vi "niRFUtil RFHS Channelizer DesignFilter_BlockSize.vi"(0 "fs":dbl=1.0, 5 "Channel Specification":T1={"fc"=0.0, "fs"=1.0, "passBW"=0.0, "stopBW"=0.0, "Rejection (dB)"=0.0, "Flags"=0, "Reserved"=0} {"Flags" items=["None"=0, "Force Fractional"=1, "Use Multistage"=2, "Use Pretrigger Data "=256, "Frequency Shift Only"=4]; "fs" format="%#_8p"; "fc" format="%#_6p"; "stopBW" format="%#_6p"; "passBW" format="%#_6p"}, 11 "error in (no error)":errorcluster) -> (4 "Filter Taps":i32, 6 "upsample":i32, 8 "downsample":dbl, 15 "error out":errorcluster)   [LabVIEW 2015, in "niRFUtil.lvlib"]
uses:
  niRFUtil.lvlib
  Includes/niRFUtil RFHS Channelizer ChannelSpecificationBase.ctl
  Includes/niRFUtil RFHS Channelizer ChannelFlags.ctl
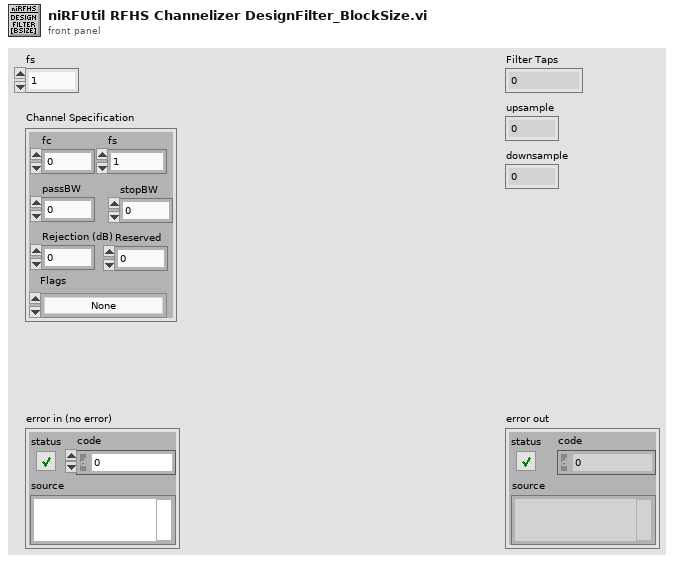
[diagram p1: front panel]
types:
  T1 = typedef "niRFUtil.lvlib/niRFUtil RFHS Channelizer ChannelSpecificationBase.ctl" = cluster{"fc":dbl, "fs":dbl, "passBW":dbl, "stopBW":dbl, "Rejection (dB)":dbl, "Flags":T2, "Reserved":i32}
  T2 = typedef "niRFUtil.lvlib/niRFUtil RFHS Channelizer ChannelFlags.ctl" = u32
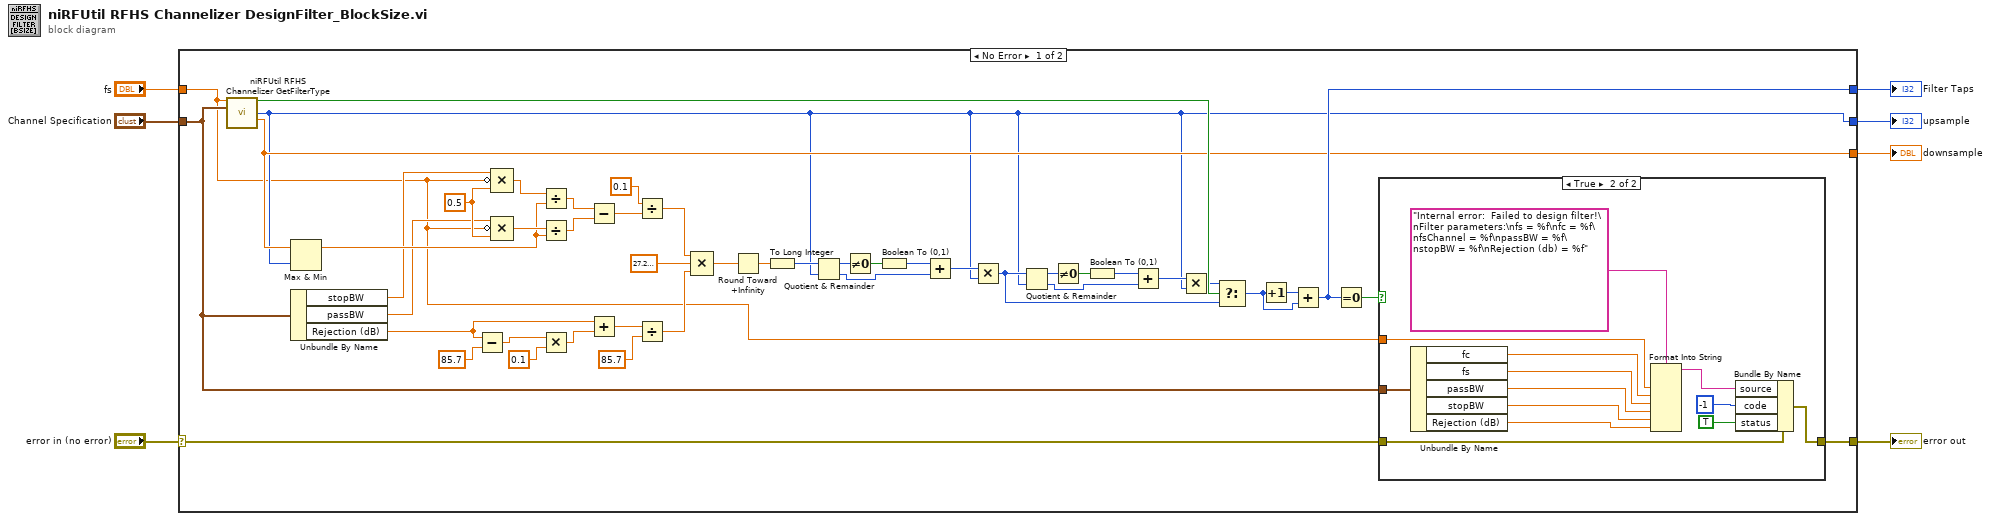
[diagram p0: block diagram]
diagram:
  n1 = case shown="No Error" "error in (no error)" {
    selector: "error in (no error)" -> [w19 w68]
    tunnel: [w21 w68] -> w7
    tunnel: "fs" -> [w8 _]
    tunnel: "Channel Specification" -> [w20 _]
    tunnel: [w17 _] -> w4
    tunnel: [w16 _] -> w2
    tunnel: [w15 _] -> w1
    frame No Error {
      w33 = 0.5 ("value")
      n2 = call "niRFUtil RFHS Channelizer GetFilterType.vi"("fs"=w8, "Channel Specification"=w20) -> ("Fractional"=w26:bool, "Upsample"=w15:i32, "Downsample"=w16:dbl)  [unwired: 10 in, 1 out]
      n3 = Max & Min(x=w16, y=w15) -> (max(x,y)=w31:dbl)  [unwired: 1 out]
      n4 = Unbundle By Name(w20) -> ("stopBW"=w14:dbl, "passBW"=w13:dbl, "Rejection (dB)"=w40:dbl)
      n5 = Subtract(x=w40, y=85.7) -> (x-y=w12:dbl)
      n6 = Compound Arithmetic op=MULTIPLY(w14, invert w8, w33) -> (w32:dbl)
      n7 = Compound Arithmetic op=MULTIPLY(w13, invert w8, w33) -> (w44:dbl)
      n8 = Divide(x=w32, y=w31) -> (x/y=w42:dbl)
      n9 = Divide(x=w44, y=w31) -> (x/y=w43:dbl)
      n10 = Multiply(x=w12, y=0.1 ("x")) -> (x*y=w47:dbl)
      n11 = Subtract(x=w42, y=w43) -> (x-y=w51:dbl)
      n12 = Add(x=w40, y=w47) -> (x+y=w46:dbl)
      n13 = Divide(x=0.1 ("y"), y=w51) -> (x/y=w45:dbl)
      n14 = Divide(x=w46, y=85.7) -> (x/y=w49:dbl)
      n15 = Compound Arithmetic op=MULTIPLY(w45, sgl 27.2 ("y"), w49) -> (w41:dbl)
      n16 = Round Toward +Infinity(x=w41) -> (ceil(x): smallest int >= x=w34:dbl)
      n17 = To Long Integer(number=w34) -> (32bit integer=w23:i32)
      n18 = Quotient & Remainder(x=w23, y=w15) -> (x-y*floor(x/y)=w39:i32, floor(x/y)=w36:i32)
      n19 = Not Equal To 0?(x=w39) -> (x != 0?=w38:bool)
      n20 = Boolean To (0,1)(Boolean=w38) -> (0, 1=w37:i16)
      n21 = Add(x=w37, y=w36) -> (x+y=w35:i32)
      n22 = Multiply(x=w35, y=w15) -> (x*y=w24:i32)
      n23 = Quotient & Remainder(x=w24, y=w15) -> (x-y*floor(x/y)=w27:i32, floor(x/y)=w10:i32)
      n24 = Not Equal To 0?(x=w27) -> (x != 0?=w28:bool)
      n25 = Boolean To (0,1)(Boolean=w28) -> (0, 1=w29:i16)
      n26 = Add(x=w29, y=w10) -> (x+y=w30:i32)
      n27 = Multiply(x=w30, y=w15) -> (x*y=w25:i32)
      n28 = Select(t=w25, s=w26, f=w24) -> (s? t:f=w9:i32)
      n29 = Increment(x=w9) -> (x+1=w18:i32)
      n30 = Add(x=w18, y=w9) -> (x+y=w17:i32)
      n31 = Equal To 0?(x=w17) -> (x = 0?=w22:bool)
      n32 = case shown="True" w22 {
        tunnel: w19 -> [w54 w67]
        tunnel: [w54 w66] -> w21
        tunnel: w8 -> [_ w61]
        tunnel: w20 -> [_ w62]
        frame False {
        }
        frame True {
          n33 = Unbundle By Name(w62) -> ("fc"=w58:dbl, "fs"=w57:dbl, "passBW"=w56:dbl, "stopBW"=w55:dbl, "Rejection (dB)"=w59:dbl)
          n34 = Format Into String(format string="Internal error:  Failed to design filter!\nFilter parameters:\nfs = %f\nfc = %f\nfsChannel = %f\npassBW = %f\nstopBW = %f\nRejection (db) = %f", w61, w58, w57, w56, w55, w59) -> (resulting string=w63:string)  [unwired: 2 in, 1 out]
          n35 = Bundle By Name(cluster=w67, "source"=w63, "code"=-1, "status"=TRUE) -> (w66:errorcluster)
        }
      }
    }
    frame Error {
    }
  }
  "error out" <- w7
  "Filter Taps" <- w4
  "downsample" <- w2
  "upsample" <- w1
